vi "DriveStright.vi"(9 "Joy Y in":dbl, 10 "Drive Stright":bool, 11 "Joy X in":dbl) -> (2 "Joy Y out":dbl, 3 "Joy X out":dbl)   [LabVIEW 2016]
uses:
  Robot Global Data.vi
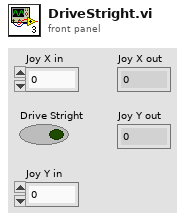
[diagram p1: front panel]
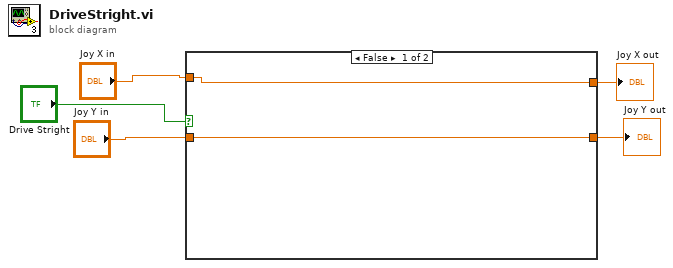
[diagram p0: block diagram]
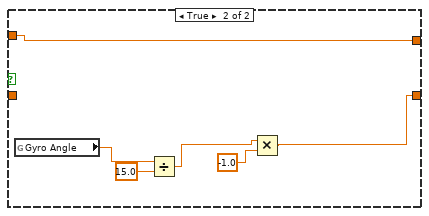
[diagram p2: hidden frame]
diagram:
  n1 = case shown="False" "Drive Stright" {
    tunnel: "Joy X in" -> [w7 w13]
    tunnel: [w7 w13] -> w3
    tunnel: [w6 w9] -> w4
    tunnel: "Joy Y in" -> [w6 _]
    frame False {
    }
    frame True {
      n2 = global read "Robot Global Data.vi" "Gyro Angle"() -> (w12:dbl)
      n3 = Divide(x=w12, y=15.0) -> (x/y=w10:dbl)
      n4 = Multiply(x=w10, y=-1.0) -> (x*y=w9:dbl)
    }
  }
  "Joy Y out" <- w4
  "Joy X out" <- w3
